vi "FunctionGenerator_Position_Control_Example.vi"() -> ()   [LabVIEW 2019]
uses:
  <vilib>/Rock Robotics/WPI/ThirdParty/JAS_Junk/TrajLib/TypeDef/X_Y_PAIR.ctl
  <vilib>/Rock Robotics/WPI/ThirdParty/JAS_Junk/TrajLib/VI/FunctionGenerator_New.vi
  <vilib>/Rock Robotics/WPI/ThirdParty/JAS_Junk/TrajLib/VI/FunctionGenerator_Calculate.vi
  <vilib>/gmath/interp.llb/Search Ordered Table.vi
  <vilib>/Rock Robotics/WPI/ThirdParty/JAS_Junk/TrajLib/Trajectory_Library.lvlib
panel:
  in  "Tab Control":T1(tab)
  out "Speed Chart":dbl(graph)
  in  "Desired Position\nFt":dbl(slide) min=0.0 max=90.0 scale=-50.0..50.0
  in  "Set Desired \nPosition to \n0 Ft":bool
  in  "Set Desired \nPosition to\n15 ft":bool
  in  "Turn on to\nuse slider\nas setpoint":bool
  out "Position Error":dbl format="%14.2f"
  out "SP, PV, CO Chart":T2(graph)
  out "In Position":bool
  out "Motor-Demand":dbl format="%14.3f"
  out "Position\nFt":dbl format="%14.2f"
  out "Setpoint\nFt":dbl format="%14.2f"
  out "Velocity Ft/Sec":dbl format="%16.1f"
  in  "Function Generator Tuning":T3[](array[typedef])=[{"X"=-8.0, "Y"=-1.0}, {"X"=-5.0, "Y"=-1.0}, {"X"=-0.06, "Y"=-0.15}, {"X"=-0.05, "Y"=0.0}, {"X"=0.05, "Y"=0.0}, {"X"=0.06, "Y"=0.15}, {"X"=5.0, "Y"=1.0}, {"X"=8.0, "Y"=1.0}] {"Y" format="%_7f"; "X" format="%_7f"}
  # "Example of Using a Function Generator for Position Control"
  # "Simulate a robot driving forward to a particular position.  A function generator is used to calculate the desired\nmotor output based on the position error.  The maximum robot speed is 8 ft/sec."
  # "Press one of the buttons \nto set the desired position.  \nThis \"target\" value is \ncalledthe \"Set Point\"."
  # "X = Position Error, Y = Motor Demand (Y could be motor speed demand)"
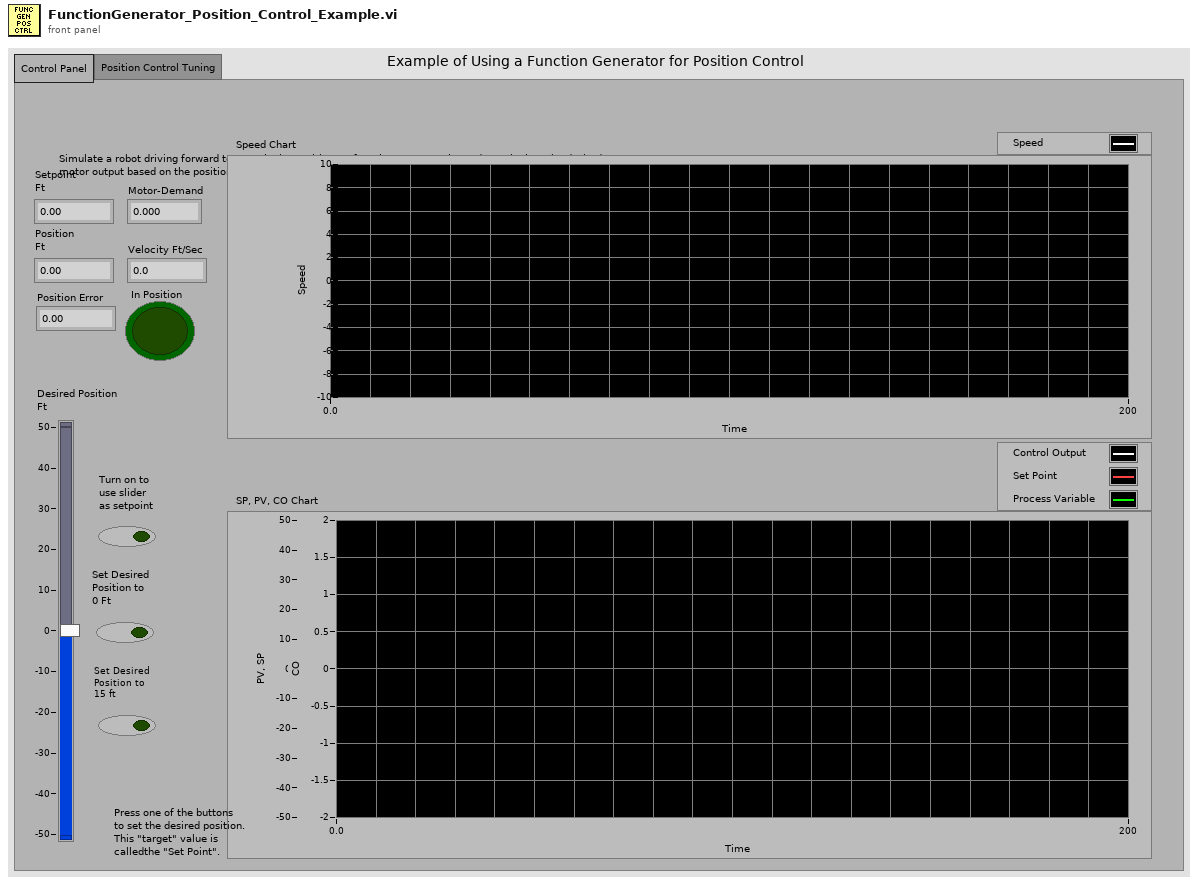
[diagram p1: front panel]
types:
  T1 = enum32{"Control Panel", "Position Control Tuning"}
  T2 = cluster{"MotorDemand":dbl, "CurrentSetpoint":dbl, "CurrentPosition":dbl}
  T3 = typedef "Trajectory_Library.lvlib/X_Y_PAIR.ctl" = cluster{"X":dbl, "Y":dbl}
  T4 = cluster{"Motor-Demand":dbl, "Setpoint\nFt":dbl, "Position\nFt":dbl}
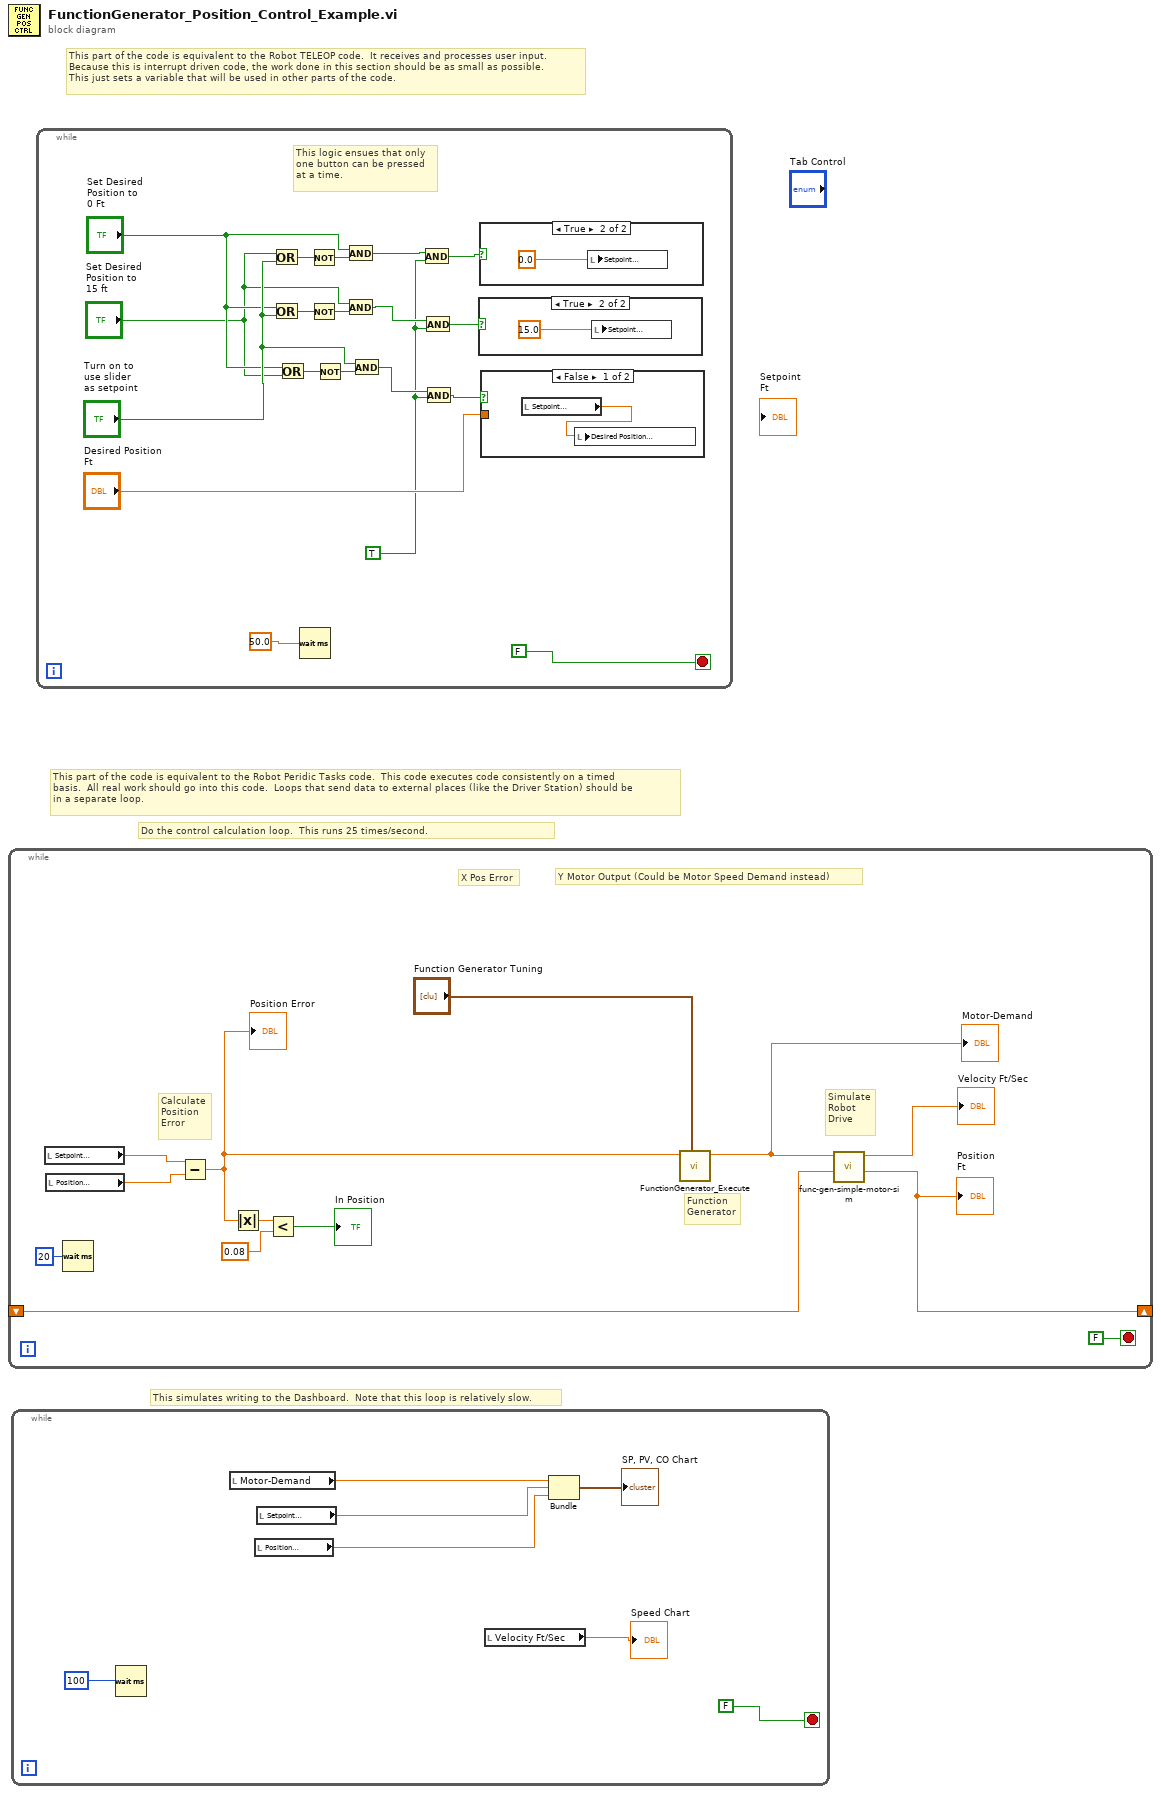
[diagram p0: block diagram]
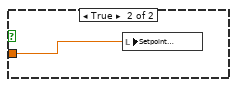
[diagram p2: hidden frame]
diagram:
  # "This simulates writing to the Dashboard.  Note that this loop is relatively slow."
  # "Do the control calculation loop.  This runs 25 times/second."
  # "This part of the code is equivalent to the Robot Peridic Tasks code.  This code executes code consistently on a timed\nbasis.  All real work should go into this code.  Loops that send data to external places (like the Driver Station) should be \nin a separate loop."
  # "This part of the code is equivalent to the Robot TELEOP code.  It receives and processes user input.\nBecause this is interrupt driven code, the work done in this section should be as small as possible.\nThis just sets a variable that will be used in other parts of the code."
  n1 = while {
    shift-right: [w10] -> _
    shift-left: _ -> [w9]
    stop <- FALSE stop-if-true
    # "Function\nGenerator"
    # "Y Motor Output (Could be Motor Speed Demand instead)"
    # "X Pos Error"
    # "Calculate\nPosition\nError"
    # "Simulate\nRobot\nDrive"
    n2 = local read "Setpoint\nFt"() -> (w8:dbl)
    n3 = local read "Position\nFt"() -> (w7:dbl)
    n4 = Wait (ms)(milliseconds to wait=u32 20) -> ()  [unwired: 1 out]
    n5 = Subtract(x=w8, y=w7) -> (x-y=w2:dbl)
    "Position Error" <- w2
    n6 = Absolute Value(x=w2) -> (abs(x)=w6:dbl)
    n7 = Less?(x=w6, y=0.08) -> (x < y?=→"In Position":bool)
    n8 = call <vilib>:"FunctionGenerator_Execute.vi"("X Y Pairs"="Function Generator Tuning", "Input Value"=w2) -> ("Output Value"=w1:dbl)  [unwired: 9 in]
    "Motor-Demand" <- w1
    n9 = call "func-gen-simple-motor-sim.vi"("Current Position Ft"=w9, "Motor-Demand"=w1) -> ("Updated Position Ft"=w10:dbl, "Velocity Ft/Sec"=→"Velocity Ft/Sec":dbl)  [unwired: 8 in]
    "Position\nFt" <- w10
  }
  n10 = while {
    stop <- FALSE stop-if-true
    n11 = Wait (ms)(milliseconds to wait=u32 100) -> ()  [unwired: 1 out]
    n12 = local read "Motor-Demand"() -> (w16:dbl)
    n13 = local read "Position\nFt"() -> (w15:dbl)
    n14 = local read "Setpoint\nFt"() -> (w18:dbl)
    n15 = local read "Velocity Ft/Sec"() -> (→"Speed Chart":dbl)
    n16 = Bundle("Motor-Demand"=w16, "Setpoint\nFt"=w18, "Position\nFt"=w15) -> (→"SP, PV, CO Chart":T4)  [unwired: 1 in]
  }
  n17 = while {
    stop <- FALSE stop-if-true
    w21 = TRUE
    # "This logic ensues that only\none button can be pressed\nat a time."
    n18 = Or(x="Set Desired \nPosition to\n15 ft", y="Turn on to\nuse slider\nas setpoint") -> (x .or. y?=w39:bool)
    n19 = Or(x="Set Desired \nPosition to \n0 Ft", y="Turn on to\nuse slider\nas setpoint") -> (x .or. y?=w37:bool)
    n20 = Or(x="Set Desired \nPosition to \n0 Ft", y="Set Desired \nPosition to\n15 ft") -> (x .or. y?=w35:bool)
    n21 = Wait (ms)(milliseconds to wait=50.0) -> ()  [unwired: 1 out]
    n22 = Not(x=w39) -> (.not. x?=w38:bool)
    n23 = Not(x=w37) -> (.not. x?=w36:bool)
    n24 = Not(x=w35) -> (.not. x?=w34:bool)
    n25 = And(x="Set Desired \nPosition to \n0 Ft", y=w38) -> (x .and. y?=w30:bool)
    n26 = And(x="Set Desired \nPosition to\n15 ft", y=w36) -> (x .and. y?=w26:bool)
    n27 = And(x="Turn on to\nuse slider\nas setpoint", y=w34) -> (x .and. y?=w25:bool)
    n28 = And(x=w30, y=w21) -> (x .and. y?=w29:bool)
    n29 = And(x=w26, y=w21) -> (x .and. y?=w28:bool)
    n30 = And(x=w25, y=w21) -> (x .and. y?=w27:bool)
    n31 = case shown="True" w28 {
      frame False {
      }
      frame True {
        n32 = local write "Setpoint\nFt"(15.0) -> ()
      }
    }
    n33 = case shown="True" w29 {
      frame False {
      }
      frame True {
        n34 = local write "Setpoint\nFt"(0.0) -> ()
      }
    }
    n35 = case shown="False" w27 {
      tunnel: "Desired Position\nFt" -> [_ w41]
      frame False {
        n36 = local read "Setpoint\nFt"() -> (w40:dbl)
        n37 = local write "Desired Position\nFt"(w40) -> ()
      }
      frame True {
        n38 = local write "Setpoint\nFt"(w41) -> ()
      }
    }
  }
